vi "Query Error.vi"(8 "error in (no error)":errorcluster, 11 "34401 in":refnum<class "34401.lvclass">) -> (0 "error out":errorcluster, 1 "Error Message":string, 2 "Error Code":i32, 3 "34401 out":refnum<class "34401.lvclass">)   [LabVIEW 2018, in "34401.lvlib" / "34401.lvclass"]
uses:
  34401.lvclass
  34401.lvclass/34401.ctl
  <instrlib>/Agilent 34401/Agilent 34401.lvlib
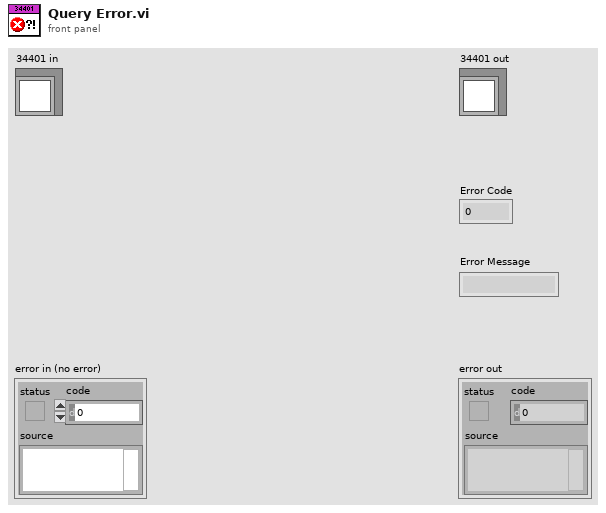
[diagram p1: front panel]
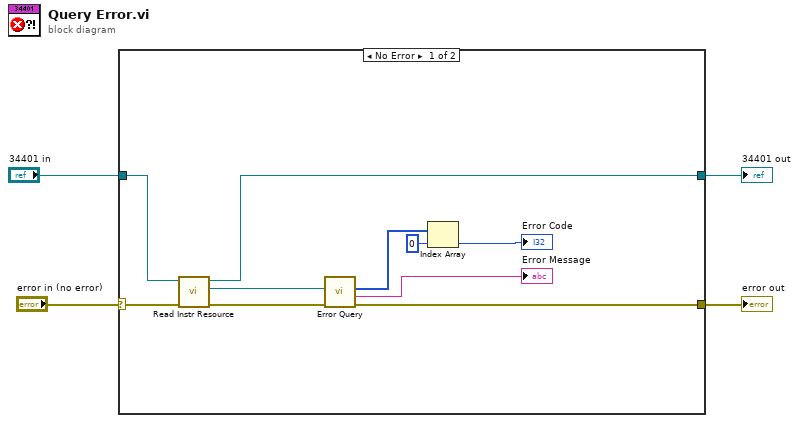
[diagram p0: block diagram]
diagram:
  n1 = case shown="No Error" "error in (no error)" {
    selector: "error in (no error)" -> [w14 w16]
    tunnel: [w5 w16] -> w3
    tunnel: [w10 w15] -> w2
    tunnel: "34401 in" -> [w13 w15]
    frame No Error {
      n2 = call "Read Instr Resource.vi"("error in (no error)"=w14, "34401 in"=w13) -> ("error out"=w12:errorcluster, "Instr Resource"=w11:refnum<visa-resource-name>, "34401 out"=w10:refnum<class "34401.lvclass">)  [unwired: 7 in]
      n3 = call <instrlib>:"Error Query.vi"("error in (no error)"=w12, "VISA resource name"=w11) -> ("error out"=w5:errorcluster, "Error Message"=→"Error Message":string, "Error Code"=w9:i32[])  [unwired: 6 in, 1 out]
      n4 = Index Array(array=w9, index=0) -> (element=→"Error Code":i32)
    }
    frame Error {
    }
  }
  "error out" <- w3
  "34401 out" <- w2
